vi "PPMS_Femto_TXT_Global_WRITE.vi"(2 "Value":i32, 3 "Property":u16(ring)=6 items=["1 - DDPCA Gain (V/A)", "2 - DDPCA Gain (V/A)", "3 - DLPVA Gain (dB)", "3 - Gain 1", "3 - Gain 2", "3 - AC/DC coupling", "3 - filter", "4 - DLPVA Gain (dB)", "4 - Gain 1", "4 - Gain 2", "4 - AC/DC coupling", "4 - filter"]) -> ()   [LabVIEW 2010]
uses:
  <vilib>/Utility/file.llb/Read From Spreadsheet File (string).vi
  <vilib>/Utility/file.llb/Write To Spreadsheet File (string).vi
panel:
  in  "file path (dialog if empty)":path=path "C:/user/patrick/PPMS_Femto/subVIs/PPMS_Femto_TXT_Global.vi.txt"
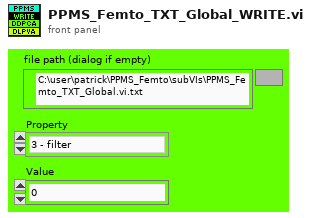
[diagram p1: front panel]
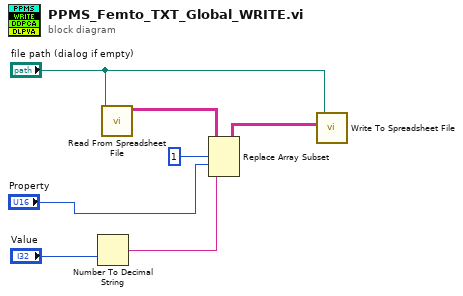
[diagram p0: block diagram]
diagram:
  n1 = Number To Decimal String(number="Value") -> (decimal integer string=w5:string)  [unwired: 1 in]
  n2 = call-poly <vilib>:"Read From Spreadsheet File.vi"("file path (dialog if empty)"="file path (dialog if empty)") -> ("all rows"=w7:string[][])  [unwired: 6 in, 4 out]
  n3 = Replace Array Subset(array=w7, new element=w5, index (row)=1, index (col)="Property") -> (w3:string[][])
  n4 = call-poly <vilib>:"Write To Spreadsheet File.vi"("2D data"=w3, "file path (dialog if empty)"="file path (dialog if empty)") -> ()  [unwired: 6 in, 1 out]
